vi "Drive Control (SubVI).vi"(7 "H Tank Disabled":bool, 8 "Buttons":bool[](array[boolean]), 9 "Joystick Axis":dbl[](array[numeric]), 10 "PID gains Slow":T1={"proportional gain (Kc)"=0.7500000000000001, "integral time (Ti, min)"=0.004, "derivative time (Td, min)"=0.0} {"derivative time (Td, min)" format="%.3f"; "integral time (Ti, min)" format="%.3f"; "proportional gain (Kc)" format="%.3f"}, 11 "PID gains Fast":T1={"proportional gain (Kc)"=0.7500000000000001, "integral time (Ti, min)"=0.001, "derivative time (Td, min)"=0.0} {"derivative time (Td, min)" format="%.3f"; "integral time (Ti, min)" format="%.3f"; "proportional gain (Kc)" format="%.3f"}) -> ()   [LabVIEW 2014]
uses:
  <vilib>/Rock Robotics/WPI/RobotDrive/WPI_RobotDriveGetSetRefNum.vi
  <vilib>/addons/control/pid/pid.llb/PID Control Input Filter (DBL).vi
  <vilib>/addons/control/pid/pid.llb/PID (DBL).vi
  <vilib>/Rock Robotics/Network Tables/SD Write Numeric Array.vi
  <vilib>/addons/control/pid/NI_PID_pid.lvlib
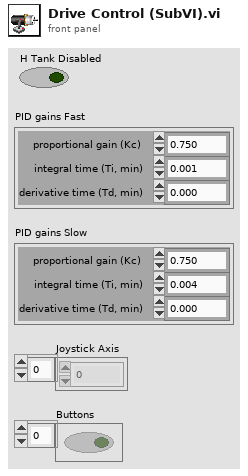
[diagram p1: front panel]
types:
  T1 = cluster{"proportional gain (Kc)":dbl, "integral time (Ti, min)":dbl, "derivative time (Td, min)":dbl}
  T2 = typedef "WPI_RobotDriveDevRef.ctl" = cluster{"DevStatus":errorcluster, "Motors[]":T3[], "Square Inputs":bool, "Max Output":dbl}
  T3 = typedef "WPI_MotorControlDeviceRef.ctl" = cluster{"DeviceStatus":errorcluster, "Type":T4, "PWM":cluster{"Controller":T5, "PWM Channel":T6, "DeadBand":T7}, "CAN":cluster{"Device Number":u8, "Control Mode":T8, "Semaphore":T9, "Max Vout":dbl, "TalonSRX Control Mode":T10}, "Invert":bool, "TransformRef":T11, "InvTransformRef":T11}
  T4 = typedef "WPI_MotorControlType.ctl" = enum16{"PWM", "CAN", "CANTalonSRX"}
  T5 = typedef "FPGA_TypedefDigitalModule.ctl" = enum16{"Controller 1"}
  T6 = typedef "FPGA_DIOPWMChannel.ctl" = enum8{"PWM 0", "PWM 1", "PWM 2", "PWM 3", "PWM 4", "PWM 5", "PWM 6", "PWM 7", "PWM 8", "PWM 9", "PWM MXP 0", "PWM MXP 1", "PWM MXP 2", "PWM MXP 3", "PWM MXP 4", "PWM MXP 5", "PWM MXP 6", "PWM MXP 7", "PWM MXP 8", "PWM MXP 9", "Invalid"}
  T7 = typedef "WPI_PWMDeadband.ctl" = cluster{"Name":string, "maxPositivePwm":i32, "minPositivePwm":i32, "centerPwm":i32, "maxNegativePwm":i32, "minNegativePwm":i32, "angularRange":u16}
  T8 = typedef "WPI_CANJaguar_ControlMode.ctl" = enum8{"Percent VBus", "Current", "Speed", "Position", "Voltage"}
  T9 = typedef "Semaphore RefNum" = refnum<k1>
  T10 = typedef "WPI_CANTalonSRX_APIControlMode.ctl" = enum8{"Percent VBus", "Speed", "Position", "Slave", "Unchanged / Invalid"}
  T11 = typedef "WPI_PWMTransform_ConPane.ctl" = refnum<vi>
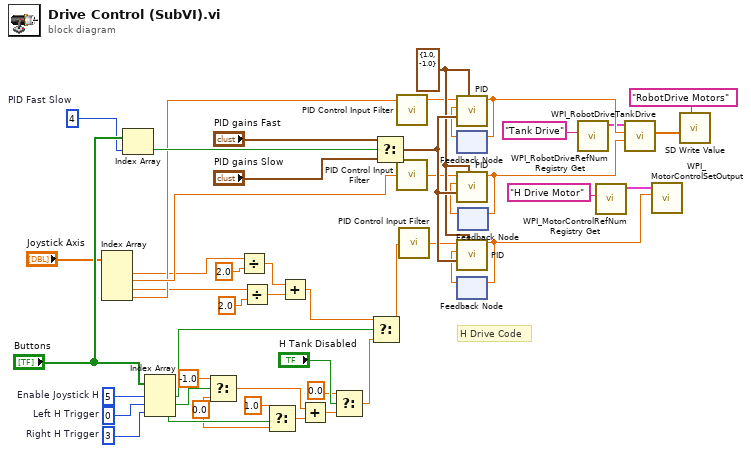
[diagram p0: block diagram]
diagram:
  w46 = 4  # PID Fast Slow
  w45 = 3  # Right H Trigger
  w41 = 0  # Left H Trigger
  w40 = 5  # Enable Joystick H
  w33 = cluster{"output high":dbl, "output low":dbl} {"output high"=1.0, "output low"=-1.0} ("output range")
  w14 = 0.0 ("t")
  # "H Drive Code"
  n1 = Index Array(array="Joystick Axis") -> (element #1=w4:dbl, element #2=w39:dbl, element #3=w5:dbl, element #4=w30:dbl)  [unwired: 4 in]
  n2 = Index Array ("H Drive Triggers")(array="Buttons", index=w46) -> (element=w48:bool)
  n3 = Index Array ("H Drive Triggers")(array="Buttons", index #1=w40, index #2=w41, index #3=w45) -> (element #1=w44:bool, element #2=w43:bool, element #3=w42:bool)
  n4 = Select(t=-1.0, s=w43, f=w14) -> (s? t:f=w13:dbl)
  n5 = Divide(x=w4, y=2.0) -> (x/y=w8:dbl)
  n6 = Divide(x=w5, y=2.0) -> (x/y=w6:dbl)
  n7 = Select(t=1.0, s=w42, f=w14) -> (s? t:f=w12:dbl)
  n8 = Add(x=w8, y=w6) -> (x+y=w34:dbl)
  n9 = Add(x=w13, y=w12) -> (x+y=w11:dbl)
  n10 = Select(t=0.0 ("f"), s="H Tank Disabled", f=w11) -> (s? t:f=w10:dbl)
  n11 = Select(t=w34, s=w44, f=w10) -> (s? t:f=w36:dbl)
  n12 = Select(t="PID gains Fast", s=w48, f="PID gains Slow") -> (s? t:f=w35:T1)
  n13 = call-poly <vilib>:"PID Control Input Filter.vi"("input"=w30) -> ("output"=w24:dbl)  [unwired: 4 in]
  n14 = call-poly <vilib>:"PID Control Input Filter.vi"("input"=w39) -> ("output"=w23:dbl)  [unwired: 4 in]
  n15 = call-poly <vilib>:"PID Control Input Filter.vi"("input"=w36) -> ("output"=w31:dbl)  [unwired: 4 in]
  n16 = feedback #1() -> (w25:dbl)  [unwired: 1 in]
  n17 = call-poly <vilib>:"PID.vi"("output range"=w33, "PID gains"=w35, "process variable"=w25, "setpoint"=w24) -> ("output"=w26:dbl)  [unwired: 6 in, 1 out]
  n18 = feedback-in #1(w26) -> ()
  n19 = feedback #2() -> (w32:dbl)  [unwired: 1 in]
  n20 = call-poly <vilib>:"PID.vi"("output range"=w33, "PID gains"=w35, "process variable"=w32, "setpoint"=w31) -> ("output"=w37:dbl)  [unwired: 6 in, 1 out]
  n21 = feedback-in #2(w37) -> ()
  n22 = feedback #3() -> (w22:dbl)  [unwired: 1 in]
  n23 = call-poly <vilib>:"PID.vi"("output range"=w33, "PID gains"=w35, "process variable"=w22, "setpoint"=w23) -> ("output"=w27:dbl)  [unwired: 6 in, 1 out]
  n24 = feedback-in #3(w27) -> ()
  n25 = call <vilib>:"WPI_RobotDriveRefNum Registry Get.vi"("refnum name"="Tank Drive") -> ("RobotDriveDevRef"=w21:T2)  [unwired: 1 in, 9 out]
  n26 = call <vilib>:"WPI_MotorControlRefNum Registry Get.vi"("refnum name"="H Drive Motor") -> ("MotorControlDevRef"=w19:T3)  [unwired: 9 in, 1 out]
  n27 = call <vilib>:"WPI_RobotDriveTankDrive.vi"("Right axis value"=w27, "Left axis value"=w26, "RobotDriveDevRef"=w21) -> ("Motor Values"=w3:dbl[])  [unwired: 6 in, 2 out]
  n28 = call <vilib>:"WPI_MotorControlSetOutput.vi"("Output"=w37, "MotorControlDevRef"=w19) -> ()  [unwired: 7 in, 3 out]
  n29 = call-poly <vilib>:"SD Write Value.vi"("Numeric Array"=w3, "Name"="RobotDrive Motors") -> ()  [unwired: 8 in, 2 out]
